vi "DigitalOutput-ScheduledDAQmxWrite.vi"(1 "ms to wait":u32, 2 "Start time":u32, 3 "data":bool[](array[boolean]), 4 "task in":refnum<k21>) -> ()   [LabVIEW 2015]
doc: "Designed to be called asynchronously, this waits [ms to wait] (as measured starting from [Start time]) and then writes the values in [data] to the task specified in [task in]."
uses:
  <vilib>/DAQmx/write.llb/DAQmx Write (Digital 1D Bool NChan 1Samp 1Line).vi
  <vilib>/DAQmx/miscellaneous.llb/DAQmx Fill In Error Info.vi
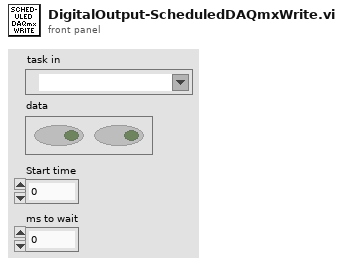
[diagram p1: front panel]
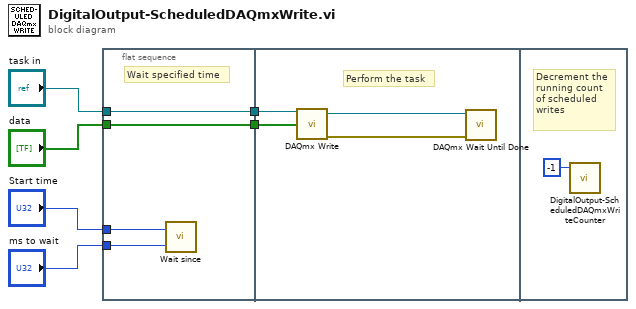
[diagram p0: block diagram]
diagram:
  n1 = flat-sequence {
    tunnel: "data" -> [w9]
    tunnel: "task in" -> [w10]
    tunnel: [w10] -> w5
    tunnel: [w9] -> w4
    tunnel: "Start time" -> [w8]
    tunnel: "ms to wait" -> [w7]
    tunnel: w5 -> [w13]
    tunnel: w4 -> [w12]
    frame #0 {
      # "Wait specified time"
      n2 = call "Wait since.vi"("ms to wait"=w7, "Start time"=w8) -> ()  [unwired: 1 in, 1 out]
    }
    frame #1 {
      # "Perform the task"
      n3 = call-poly <vilib>:"DAQmx Write.vi"("task/channels in"=w13, "data"=w12) -> ("task out"=w14:refnum<k21>, "error out"=w11:errorcluster)  [unwired: 11 in, 1 out]
      n4 = call <vilib>:"DAQmx Wait Until Done.vi"("task/channels in"=w14, "error in"=w11) -> ()  [unwired: 12 in, 2 out]
    }
    frame #2 {
      # "Decrement the\nrunning count\nof scheduled\nwrites"
      n5 = call "DigitalOutput-ScheduledDAQmxWriteCounter.vi"("Change in count"=i16 -1) -> ()  [unwired: 3 in, 2 out]
    }
  }
